vi "qmeter_graph.vi"() -> ()   [LabVIEW 2009]
panel:
  out "XY Graph":cluster{"Y":dbl[], "Y":dbl[]}[](graph)
  in  "stop (F)":bool
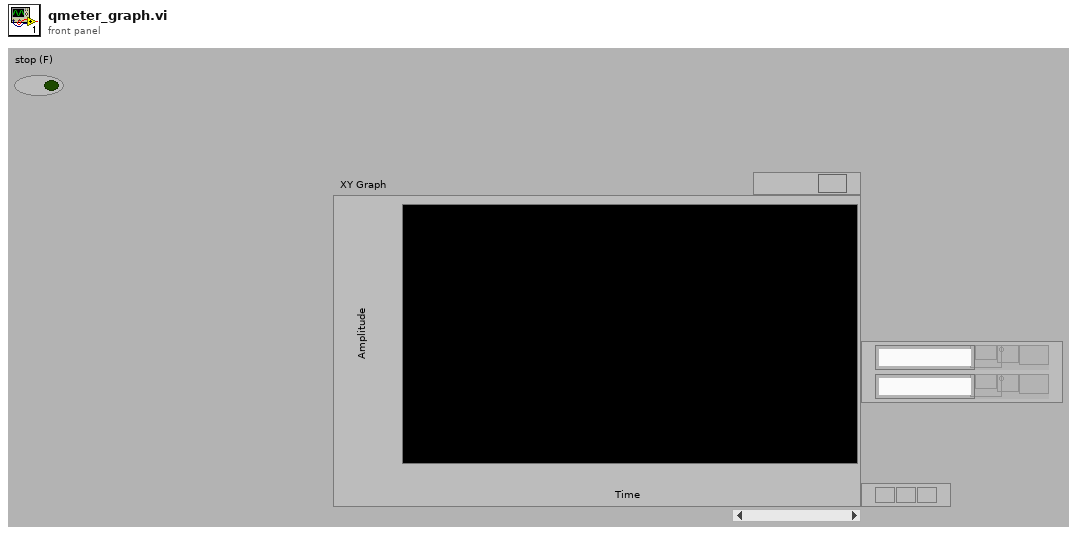
[diagram p1: front panel]
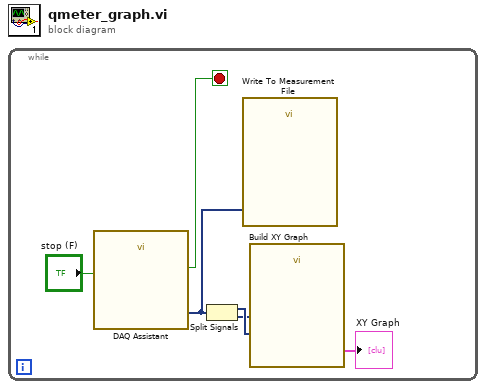
[diagram p0: block diagram]
diagram:
  n1 = while {
    stop <- w5 stop-if-true
    n2 = call "DAQ Assistant"("stop (F)"="stop (F)") -> ("data"=w1:dynamicdata, "stopped"=w5:bool)  [unwired: 15 in, 2 out]
    n3 = Split Signals(w1) -> (w3:dynamicdata, w2:dynamicdata)  [unwired: 2 in]
    n4 = call "Write To Measurement File"("Signals"=w1) -> ()  [unwired: 16 in, 3 out]
    n5 = call "Build XY Graph"("Y Input"=w3, "X Input"=w2) -> ("XY Graph"=→"XY Graph":cluster{"Y":dbl[], "Y":dbl[]}[])  [unwired: 8 in, 1 out]
  }
